vi "Control_Panel_Globals.vi"() -> ()   [LabVIEW 2019]
uses:
  Subsystems/Control_Panel/Control_Panel_Cluster.ctl
panel:
  in  "Control_Panel":string="Control_Panel"
  in  "Control_Panel_Execute_Notifier":refnum<notifier>
  in  "Control_Panel_Set_Notifier":refnum<notifier>
  in  "Control_Panel_Execute_Ref":string="Control_Panel_Execute_Ref"
  in  "Control_Panel_Set_Ref":string="Control_Panel_Set_Ref"
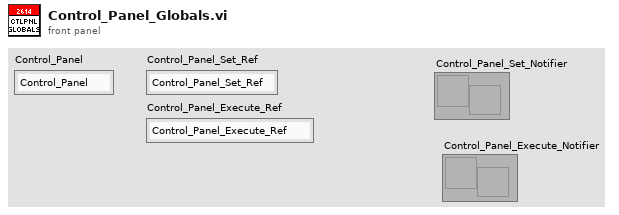
[diagram p1: front panel]
diagram:
